vi "Get_Total_Time.vi"(1 "Input Sequence":cluster{string, string[], dbl[], dbl}[](array[cluster])) -> (0 "Total Time":dbl)   [LabVIEW 2011]
doc: "This VI sums all the time values for every event in the \"Input Sequence\"."
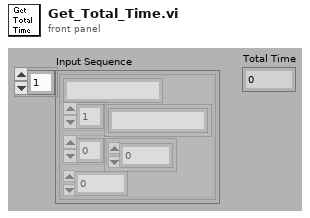
[diagram p1: front panel]
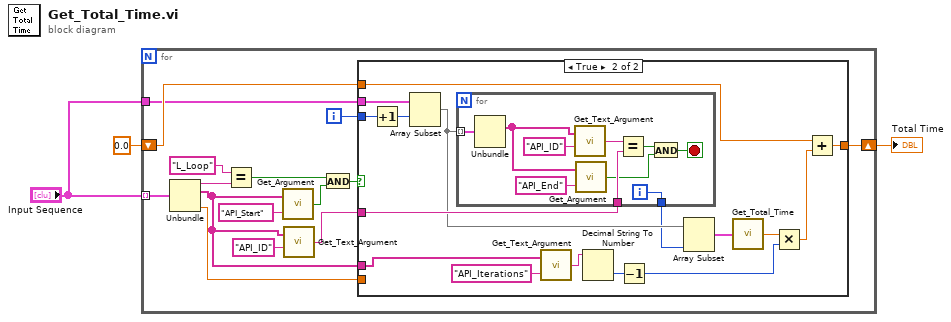
[diagram p0: block diagram]
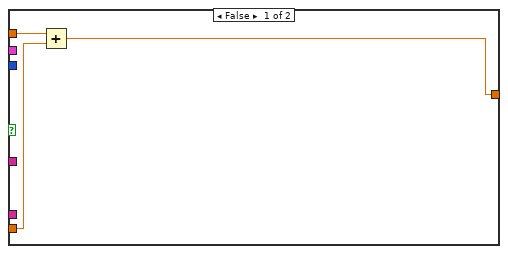
[diagram p2: hidden frame]
diagram:
  n1 = for {
    shift-right: [w13] -> w2
    shift-left: 0.0 -> [w15]
    tunnel: "Input Sequence" -> [w18] mode=indexing
    tunnel: "Input Sequence" -> [w8]
    i -> [w7]
    n2 = Unbundle(w18) -> (w17:string, w5:string[], w14:dbl)  [unwired: 1 out]
    n3 = Equal?(x="L_Loop", y=w17) -> (x = y?=w9:bool)
    n4 = call "Get_Argument.vi"("Argument"="API_Start", "Argument List"=w5) -> ("Enabled"=w10:bool)
    n5 = call "Get_Text_Argument.vi"("Argument"="API_ID", "Argument List"=w5) -> ("Text"=w4:string)
    n6 = And(x=w9, y=w10) -> (x .and. y?=w11:bool)
    n7 = case shown="True" w11 {
      tunnel: w15 -> [w20 w22]
      tunnel: w14 -> [w21 _]
      tunnel: [w19 w23] -> w13
      tunnel: w5 -> [_ w37]
      tunnel: w8 -> [_ w33]
      tunnel: w7 -> [_ w32]
      tunnel: w4 -> [_ w30]
      frame False {
        n8 = Add(x=w20, y=w21) -> (x+y=w19:dbl)
      }
      frame True {
        n9 = Increment(x=w32) -> (x+1=w31:i32)
        n10 = Array Subset(array=w33, index=w31) -> (w29:cluster{string, string[], dbl[], dbl}[])  [unwired: 1 in]
        n11 = for {
          tunnel: w29 -> [w47] mode=indexing
          tunnel: w30 -> [w44]
          tunnel: [w38] -> w28
          i -> [w38]
          stop <- w39 stop-if-true
          n12 = Unbundle(w47) -> (w42:string[])  [unwired: 3 out]
          n13 = call "Get_Text_Argument.vi"("Argument"="API_ID", "Argument List"=w42) -> ("Text"=w45:string)
          n14 = call "Get_Argument.vi"("Argument"="API_End", "Argument List"=w42) -> ("Enabled"=w40:bool)
          n15 = Equal?(x=w45, y=w44) -> (x = y?=w41:bool)
          n16 = And(x=w41, y=w40) -> (x .and. y?=w39:bool)
        }
        n17 = call "Get_Text_Argument.vi"("Argument"="API_Iterations", "Argument List"=w37) -> ("Text"=w35:string)
        n18 = Decimal String To Number(string=w35) -> (number=w34:i32)  [unwired: 2 in, 1 out]
        n19 = Decrement(x=w34) -> (x-1=w25:i32)
        n20 = Array Subset(array=w29, length=w28) -> (w27:cluster{string, string[], dbl[], dbl}[])  [unwired: 1 in]
        n21 = call "Get_Total_Time.vi"("Input Sequence"=w27) -> ("Total Time"=w26:dbl)
        n22 = Multiply(x=w26, y=w25) -> (x*y=w24:dbl)
        n23 = Add(x=w22, y=w24) -> (x+y=w23:dbl)
      }
    }
  }
  "Total Time" <- w2
